vi "TetroInfoCreation.vi"() -> (1 "TetroInfo Output":T1)   [LabVIEW 2026]
doc: "This Logic VI stores and randomly selects one of the available tetroInfos."
uses:
  02_StateMachine/GameTetrominoInformationTypeDef.ctl
  <vilib>/numeric/Random Number (Range) U64.vi
  <vilib>/numeric/sub_Random U32.vi
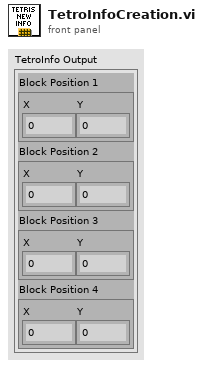
[diagram p1: front panel]
types:
  T1 = typedef "GameTetrominoInformationTypeDef.ctl" = cluster{"Block Position 1":cluster{"X":i32, "Y":i32}, "Block Position 2":cluster{"X":i32, "Y":i32}, "Block Position 3":cluster{"X":i32, "Y":i32}, "Block Position 4":cluster{"X":i32, "Y":i32}}
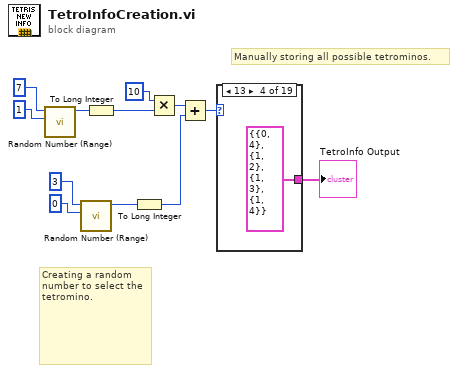
[diagram p0: block diagram]
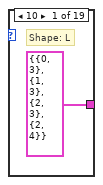
[diagram p2: hidden frame]
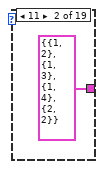
[diagram p3: hidden frame]
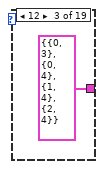
[diagram p4: hidden frame]
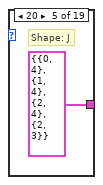
[diagram p5: hidden frame]
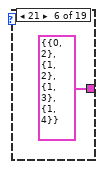
[diagram p6: hidden frame]
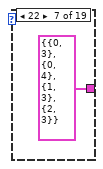
[diagram p7: hidden frame]
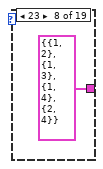
[diagram p8: hidden frame]
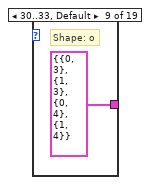
[diagram p9: hidden frame]
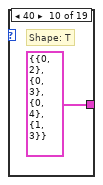
[diagram p10: hidden frame]
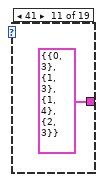
[diagram p11: hidden frame]
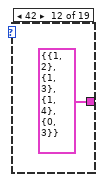
[diagram p12: hidden frame]
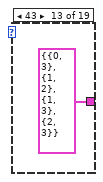
[diagram p13: hidden frame]
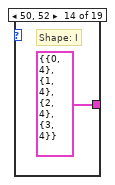
[diagram p14: hidden frame]
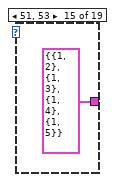
[diagram p15: hidden frame]
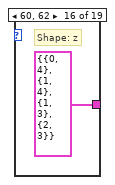
[diagram p16: hidden frame]
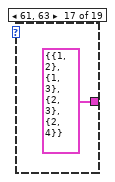
[diagram p17: hidden frame]
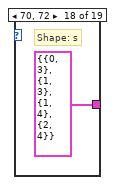
[diagram p18: hidden frame]
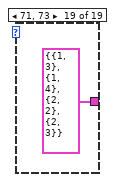
[diagram p19: hidden frame]
diagram:
  # "Manually storing all possible tetrominos."
  # "Creating a random number to select the tetromino."
  n1 = call-poly <vilib>:"Random Number (Range).vi"("lower bound (0)"=u64 1, "upper bound (100)"=u64 7) -> ("number"=w9:u64)  [unwired: 9 in]
  n2 = call-poly <vilib>:"Random Number (Range).vi"("lower bound (0)"=u64 0, "upper bound (100)"=u64 3) -> ("number"=w4:u64)  [unwired: 9 in]
  n3 = To Long Integer(number=w9) -> (32bit integer=w8:i32)
  n4 = To Long Integer(number=w4) -> (32bit integer=w2:i32)
  n5 = Multiply(x=10, y=w8) -> (x*y=w3:i32)
  n6 = Add(x=w3, y=w2) -> (x+y=w1:i32)
  n7 = case shown="13" w1 {
    tunnel: [T1 {"Block Position 1"={"X"=0, "Y"=3}, "Block Position 2"={"X"=1, "Y"=3}, "Block Position 3"={"X"=2, "Y"=3}, "Block Position 4"={"X"=2, "Y"=4}} ("TetroInfo") T1 {"Block Position 1"={"X"=1, "Y"=2}, "Block Position 2"={"X"=1, "Y"=3}, "Block Position 3"={"X"=1, "Y"=4}, "Block Position 4"={"X"=2, "Y"=2}} ("TetroInfo") T1 {"Block Position 1"={"X"=0, "Y"=3}, "Block Position 2"={"X"=0, "Y"=4}, "Block Position 3"={"X"=1, "Y"=4}, "Block Position 4"={"X"=2, "Y"=4}} ("TetroInfo") T1 {"Block Position 1"={"X"=0, "Y"=4}, "Block Position 2"={"X"=1, "Y"=2}, "Block Position 3"={"X"=1, "Y"=3}, "Block Position 4"={"X"=1, "Y"=4}} ("TetroInfo") T1 {"Block Position 1"={"X"=0, "Y"=4}, "Block Position 2"={"X"=1, "Y"=4}, "Block Position 3"={"X"=2, "Y"=4}, "Block Position 4"={"X"=2, "Y"=3}} ("TetroInfo") T1 {"Block Position 1"={"X"=0, "Y"=2}, "Block Position 2"={"X"=1, "Y"=2}, "Block Position 3"={"X"=1, "Y"=3}, "Block Position 4"={"X"=1, "Y"=4}} ("TetroInfo") T1 {"Block Position 1"={"X"=0, "Y"=3}, "Block Position 2"={"X"=0, "Y"=4}, "Block Position 3"={"X"=1, "Y"=3}, "Block Position 4"={"X"=2, "Y"=3}} ("TetroInfo") T1 {"Block Position 1"={"X"=1, "Y"=2}, "Block Position 2"={"X"=1, "Y"=3}, "Block Position 3"={"X"=1, "Y"=4}, "Block Position 4"={"X"=2, "Y"=4}} ("TetroInfo") T1 {"Block Position 1"={"X"=0, "Y"=3}, "Block Position 2"={"X"=1, "Y"=3}, "Block Position 3"={"X"=0, "Y"=4}, "Block Position 4"={"X"=1, "Y"=4}} ("TetroInfo") T1 {"Block Position 1"={"X"=0, "Y"=2}, "Block Position 2"={"X"=0, "Y"=3}, "Block Position 3"={"X"=0, "Y"=4}, "Block Position 4"={"X"=1, "Y"=3}} ("TetroInfo") T1 {"Block Position 1"={"X"=0, "Y"=3}, "Block Position 2"={"X"=1, "Y"=3}, "Block Position 3"={"X"=1, "Y"=4}, "Block Position 4"={"X"=2, "Y"=3}} ("TetroInfo") T1 {"Block Position 1"={"X"=1, "Y"=2}, "Block Position 2"={"X"=1, "Y"=3}, "Block Position 3"={"X"=1, "Y"=4}, "Block Position 4"={"X"=0, "Y"=3}} ("TetroInfo") T1 {"Block Position 1"={"X"=0, "Y"=3}, "Block Position 2"={"X"=1, "Y"=2}, "Block Position 3"={"X"=1, "Y"=3}, "Block Position 4"={"X"=2, "Y"=3}} ("TetroInfo") T1 {"Block Position 1"={"X"=0, "Y"=4}, "Block Position 2"={"X"=1, "Y"=4}, "Block Position 3"={"X"=2, "Y"=4}, "Block Position 4"={"X"=3, "Y"=4}} ("TetroInfo") T1 {"Block Position 1"={"X"=1, "Y"=2}, "Block Position 2"={"X"=1, "Y"=3}, "Block Position 3"={"X"=1, "Y"=4}, "Block Position 4"={"X"=1, "Y"=5}} ("TetroInfo") T1 {"Block Position 1"={"X"=0, "Y"=4}, "Block Position 2"={"X"=1, "Y"=4}, "Block Position 3"={"X"=1, "Y"=3}, "Block Position 4"={"X"=2, "Y"=3}} ("TetroInfo") T1 {"Block Position 1"={"X"=1, "Y"=2}, "Block Position 2"={"X"=1, "Y"=3}, "Block Position 3"={"X"=2, "Y"=3}, "Block Position 4"={"X"=2, "Y"=4}} ("TetroInfo") T1 {"Block Position 1"={"X"=0, "Y"=3}, "Block Position 2"={"X"=1, "Y"=3}, "Block Position 3"={"X"=1, "Y"=4}, "Block Position 4"={"X"=2, "Y"=4}} ("TetroInfo") T1 {"Block Position 1"={"X"=1, "Y"=3}, "Block Position 2"={"X"=1, "Y"=4}, "Block Position 3"={"X"=2, "Y"=2}, "Block Position 4"={"X"=2, "Y"=3}} ("TetroInfo")] -> w12
    frame 10 {
      # "Shape: L"
    }
    frame 11 {
    }
    frame 12 {
    }
    frame 13 {
    }
    frame 20 {
      # "Shape: J"
    }
    frame 21 {
    }
    frame 22 {
    }
    frame 23 {
    }
    frame 30..33, Default {
      # "Shape: o"
    }
    frame 40 {
      # "Shape: T"
    }
    frame 41 {
    }
    frame 42 {
    }
    frame 43 {
    }
    frame 50, 52 {
      # "Shape: I"
    }
    frame 51, 53 {
    }
    frame 60, 62 {
      # "Shape: z"
    }
    frame 61, 63 {
    }
    frame 70, 72 {
      # "Shape: s"
    }
    frame 71, 73 {
    }
  }
  "TetroInfo Output" <- w12
